vi "Core Action.vi"(8 "error in (no error)":errorcluster, 10 "SECS-II Class":refnum<class "SECS-II Class.lvclass">, 11 "31-Host Requests Time Value from Equipment in":refnum<class "31-Host Requests Time Value from Equipment.lvclass">) -> (0 "error out":errorcluster, 2 "SECS-II Class Out":refnum<class "SECS-II Class.lvclass">, 3 "31-Host Requests Time Value from Equipment out":refnum<class "31-Host Requests Time Value from Equipment.lvclass">)   [LabVIEW 2020, in "SECS Scenarios.lvlib" / "31-Host Requests Time Value from Equipment.lvclass"]
uses:
  31-Host Requests Time Value from Equipment.lvclass
  D:/Dropbox/SECS/SECS_GEM v1.1.0/Com/SECS Scenarios/Scenarios Class/Scenarios Class.lvclass
  SECS Communication/SECS-II Class/SECS-II Class.lvclass
  SECS Communication/S2 Message Class/S2 Message Class.lvclass
  D:/Dropbox/SECS/SECS_GEM v1.1.0/Com/SECS Communication/SECS-II Class/SECS-II Class.lvclass
  Scenarios Class/Reply State.ctl
  Scenarios Class/Scenarios Class.lvclass/Scenarios Class.ctl
  Scenarios Class/Write Reply State.vi
  Scenarios Class/Read HSMS Class.vi
  SECS Communication/HSMS Class/HSMS Class.lvclass
  Scenarios Class/Scenarios Class.lvclass
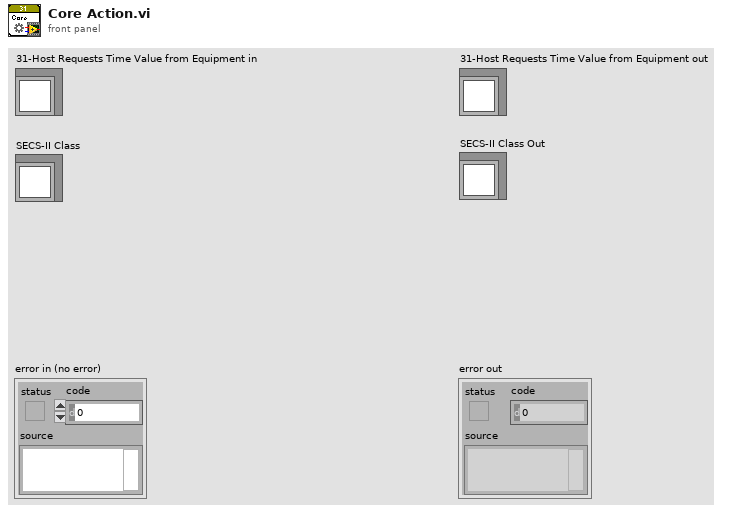
[diagram p1: front panel]
types:
  T1 = typedef "SECS Scenarios.lvlib/Scenarios Class.lvclass/Reply State.ctl" = enum16{"OK", "Illegal Data", "Unknown Stream", "Unknown Function", "Off-Line", "T3 Timeout", "Inner-Timeout"}
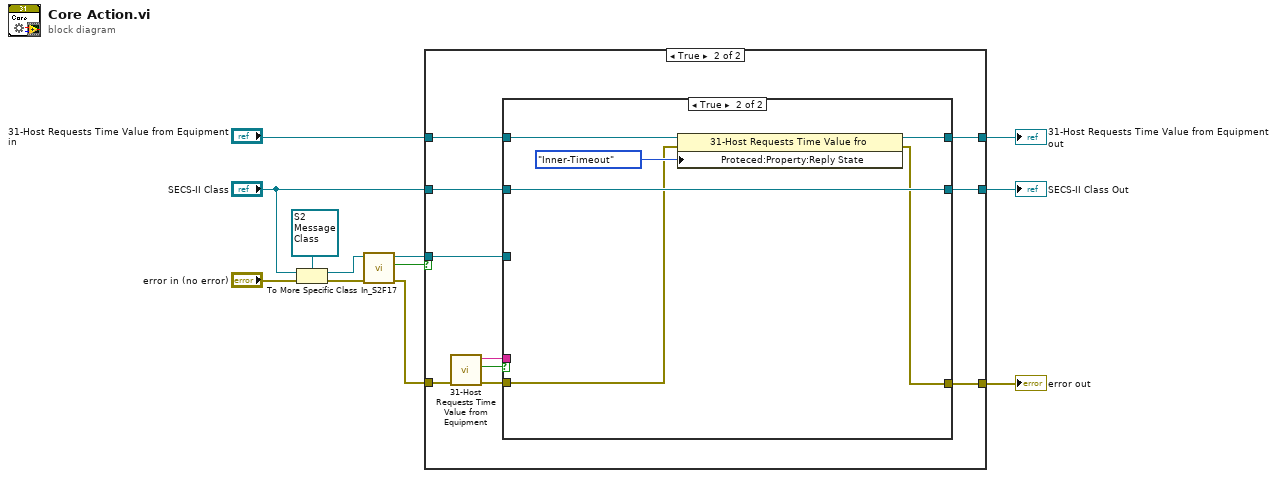
[diagram p0: block diagram]
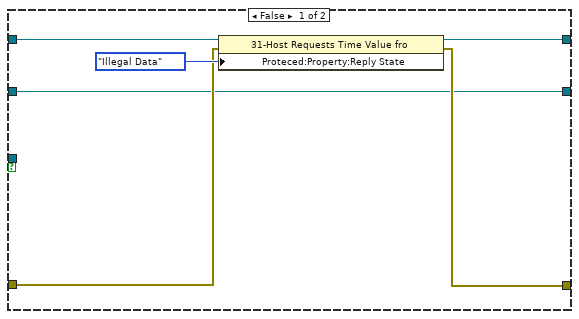
[diagram p2: hidden frame]
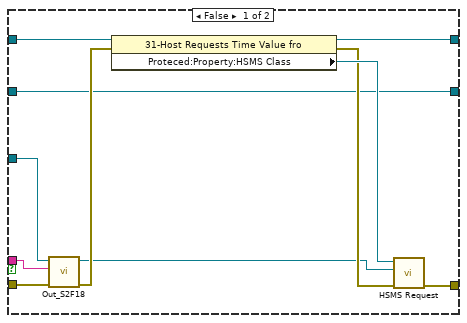
[diagram p3: hidden frame]
diagram:
  n1 = To More Specific Class(target class=refnum<class "S2 Message Class.lvclass"> refnum ("SECS Communication.lvlib:S2 Message Class.lvclass"), reference="SECS-II Class", error in="error in (no error)") -> (specific class reference=w11:refnum<class "S2 Message Class.lvclass">, error out=w12:errorcluster)
  n2 = call "In_S2F17.vi"("error in (no error)"=w12, "S2 Message Class in"=w11) -> ("error out"=w10:errorcluster, "OK?"=w5:bool, "S2 Message Class out"=w9:refnum<class "S2 Message Class.lvclass">)  [unwired: 7 in]
  n3 = case shown="True" w5 {
    tunnel: w10 -> [w15 w28]
    tunnel: w9 -> [_ w27]
    tunnel: "31-Host Requests Time Value from Equipment in" -> [w18 w24]
    tunnel: [w14 w22] -> w4
    tunnel: [w17 w21] -> w3
    tunnel: "SECS-II Class" -> [w13 w20]
    tunnel: [w13 w19] -> w1
    frame False {
      n4 = property class="31-Host Requests Time Value fro"(reference=w18, error in=w15, "Proteced:Property:Reply State"=Reply_State."Illegal Data" ("Reply State")) -> (reference out=w17:refnum<class "31-Host Requests Time Value from Equipment.lvclass">, error out=w14:errorcluster)
    }
    frame True {
      n5 = call "31-Host Requests Time Value from Equipment.vi"("error in (no error)"=w28) -> ("error out"=w26:errorcluster, "Timeout?"=w25:bool, "Time"=w23:string)  [unwired: 8 in]
      n6 = case shown="True" w25 {
        tunnel: w24 -> [w39 w43]
        tunnel: w27 -> [w35 _]
        tunnel: [w31 w40] -> w22
        tunnel: [w36 w42] -> w21
        tunnel: w26 -> [w32 w41]
        tunnel: w23 -> [w30 _]
        tunnel: w20 -> [w29 w45]
        tunnel: [w29 w45] -> w19
        frame False {
          n7 = call "Out_S2F18.vi"("error in (no error)"=w32, "Time"=w30, "S2 Message Class in"=w35) -> ("error out"=w34:errorcluster, "S2 Message Class out"=w33:refnum<class "S2 Message Class.lvclass">)  [unwired: 7 in]
          n8 = property class="31-Host Requests Time Value fro"(reference=w39, error in=w34) -> (reference out=w36:refnum<class "31-Host Requests Time Value from Equipment.lvclass">, error out=w37:errorcluster, "Proteced:Property:HSMS Class"=w38:refnum<class "HSMS Class.lvclass">)
          n9 = call "HSMS Request.vi"("error in (no error)"=w37, "SECS-II Class In"=w33, "HSMS Class in"=w38) -> ("error out"=w31:errorcluster)  [unwired: 7 in, 1 out]
        }
        frame True {
          n10 = property class="31-Host Requests Time Value fro"(reference=w43, error in=w41, "Proteced:Property:Reply State"=Reply_State."Inner-Timeout" ("Reply State")) -> (reference out=w42:refnum<class "31-Host Requests Time Value from Equipment.lvclass">, error out=w40:errorcluster)
        }
      }
    }
  }
  "error out" <- w4
  "31-Host Requests Time Value from Equipment out" <- w3
  "SECS-II Class Out" <- w1
